vi "Write Self Actor Attributes.vi"(10 "Self Actor Attributes":T1, 11 "Base Actor in":refnum<class "Base Actor.lvclass">) -> (3 "Base Actor out":refnum<class "Base Actor.lvclass">)   [LabVIEW 2020, in "jettl.lvlib" / "Base jettl Actor.lvlib" / "Base Actor.lvlib" / "Base Actor.lvclass"]
uses:
  Base Actor.lvclass
  Base Actor.lvclass/Base Actor.ctl
  Msg/Msg.lvclass
  Msg Input/Msg Input.lvclass
  Msg Output/Msg Output.lvclass
  Actor Attributes.ctl
  jettl.lvlib
  Unified Layer.ctl
  Msgs.ctl
  Msg Attributes.ctl
  Teller.ctl
  Relation.ctl
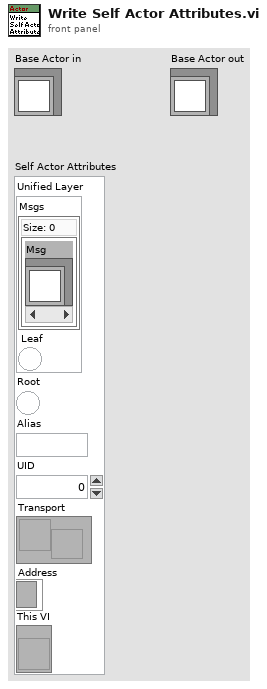
[diagram p1: front panel]
types:
  T1 = typedef "jettl.lvlib/Actor Attributes.ctl" = cluster{"Unified Layer":T2, "Root":bool, "Alias":string, "UID":i32, "Transport":refnum<user-event>, "Address":refnum<event-registration>, "This VI":refnum<vi>}
  T2 = typedef "jettl.lvlib/Unified Layer.ctl" = cluster{"Msgs":T3, "Leaf":bool}
  T3 = typedef "jettl.lvlib/Msgs.ctl" = set{refnum<class "Msg.lvclass">}
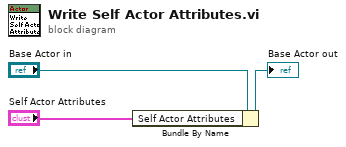
[diagram p0: block diagram]
diagram:
  n1 = Bundle By Name(cluster="Base Actor in", "Self Actor Attributes"="Self Actor Attributes") -> (→"Base Actor out":refnum<class "Base Actor.lvclass">)
